vi "Main-RC.vi"() -> ()   [LabVIEW 2020]
uses:
  States.ctl
  <vilib>/measure/NI_MAPro.lvlib
  <vilib>/measure/matone.llb/Extract Single Tone Information 1 Chan.vi
  <vilib>/Analysis/NI_AALBase.lvlib
  <vilib>/Analysis/NI_AALPro.lvlib
  <vilib>/Analysis/6fits.llb/Confidence Interval (Exp).vi
  <vilib>/Analysis/baseanly.llb/Mean (DBL).vi
  <vilib>/DAQmx/read.llb/DAQmx Read (Analog 1D Wfm NChan NSamp).vi
  DAQmx_Parameters.ctl
  DAQmx_Channels.ctl
panel:
  in  "N_offset":i32 caption="last points"
  in  "Subtract":bool caption="Subtract mean of"
  out "DRC":dbl caption="us"
  out "RC=":dbl
  out "Fit XY Graph":cluster{dbl[], "Best Exponential Fit":dbl[]}[](graph) caption="Exponential Fit"
  in  "On/Off":bool
  in  "Fit Channel":u16(ring) caption="Analyse Channel" items=["Primo", "Secondo", "Terzo"]
  in  "ClearGraph":bool
  out "Freq Analisys":cluster{"X":dbl, "Y":dbl}[](graph) caption="Frequency Analysis"
  in  "Freq Chn":u16(ring) caption="Analyse Channel" items=["Primo", "Secondo", "Terzo"]
  out "data":waveform(dbl)[](graph) caption="DAQ Graphs"
  in  "DAQ Channels":T1=[{"DAQmx Physical"="", "Logic Name"="V_S", "Min Value"=-10.0, "Max Value"=10.0}, {"DAQmx Physical"="", "Logic Name"="V_C", "Min Value"=-10.0, "Max Value"=10.0}, {"DAQmx Physical"="", "Logic Name"="V_R", "Min Value"=-10.0, "Max Value"=10.0}]
  in  "DAQ Params":T2={"Trigger Level"=1.0, "Trigger Slope"=10280, "Sample Rate"=10000.0, "N Samples"=300} {"Trigger Slope" items=["Rising"=10280, "Falling"=10171]; "Trigger Level" scale=0.0..10.0}
  in  "FIT":bool caption="+ / -"
  in  "DAQ":bool
  in  "Stop":bool
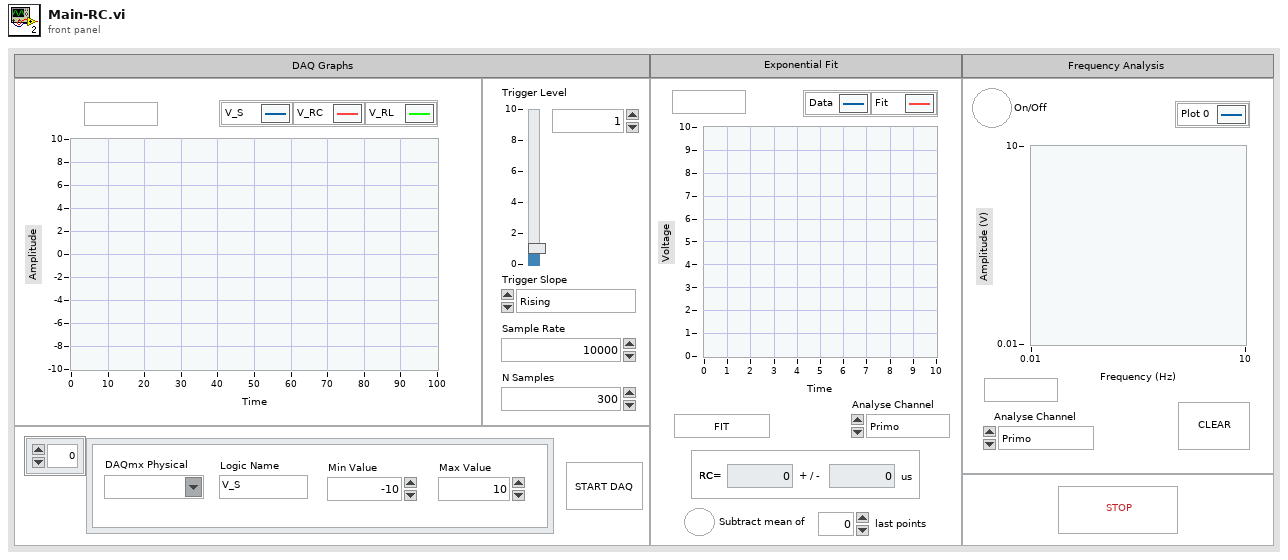
[diagram p1: front panel]
types:
  T1 = typedef "DAQmx_Channels.ctl" = cluster{"DAQmx Physical":tag, "Logic Name":string, "Min Value":dbl, "Max Value":dbl}[]
  T2 = typedef "DAQmx_Parameters.ctl" = cluster{"Trigger Level":dbl, "Trigger Slope":i32, "Sample Rate":dbl, "N Samples":i32}
  T3 = cluster{"detected frequency":dbl, "detected amplitude":dbl}[]
  T4 = typedef "States.ctl" = enum16{"Idle", "Acquire", "Fit", "Stop"}
  T5 = cluster{"detected frequency":dbl, "detected amplitude":dbl}
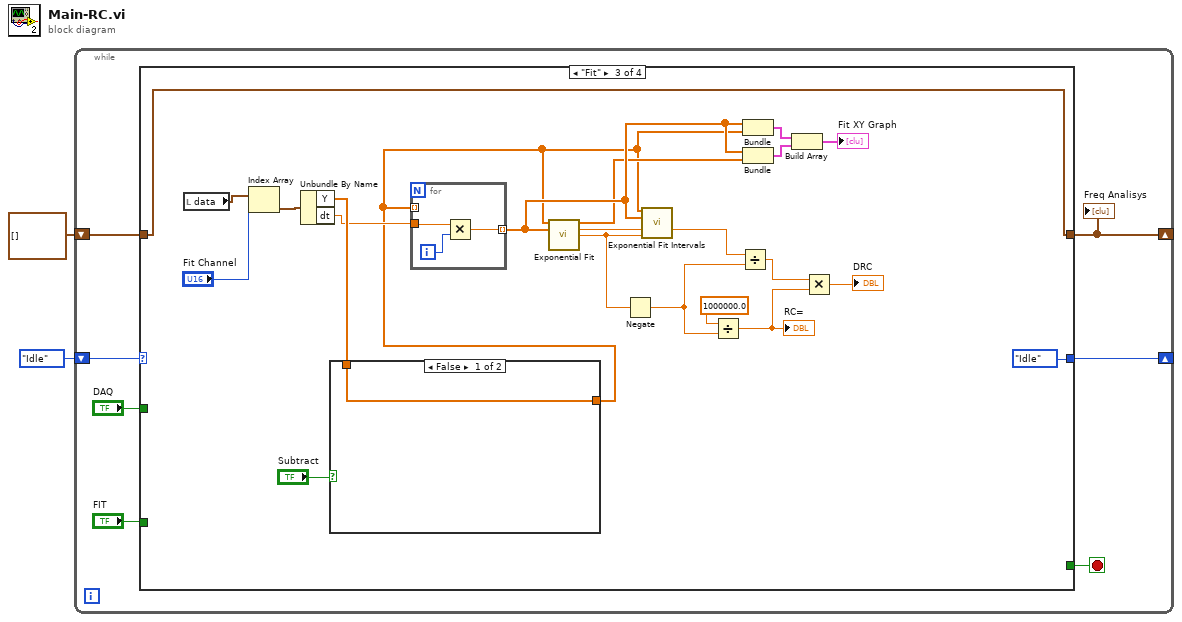
[diagram p0: block diagram]
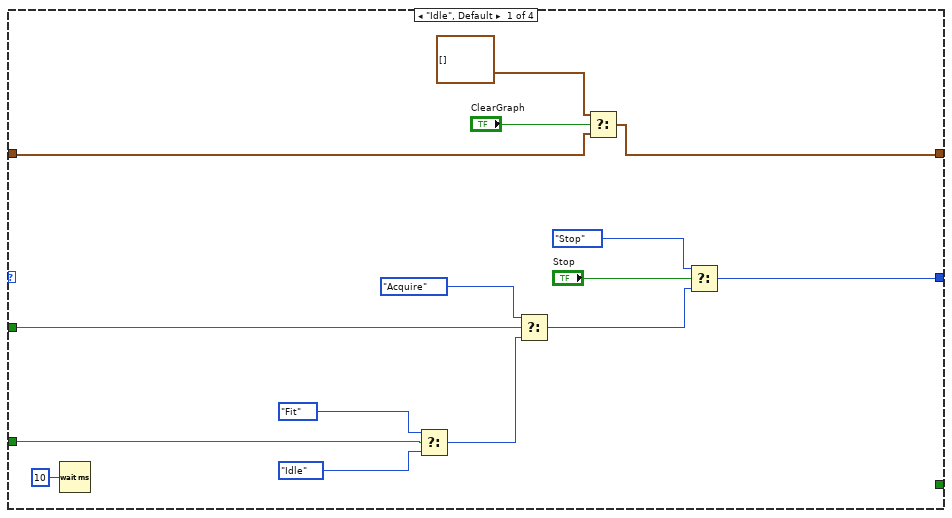
[diagram p2: hidden frame]
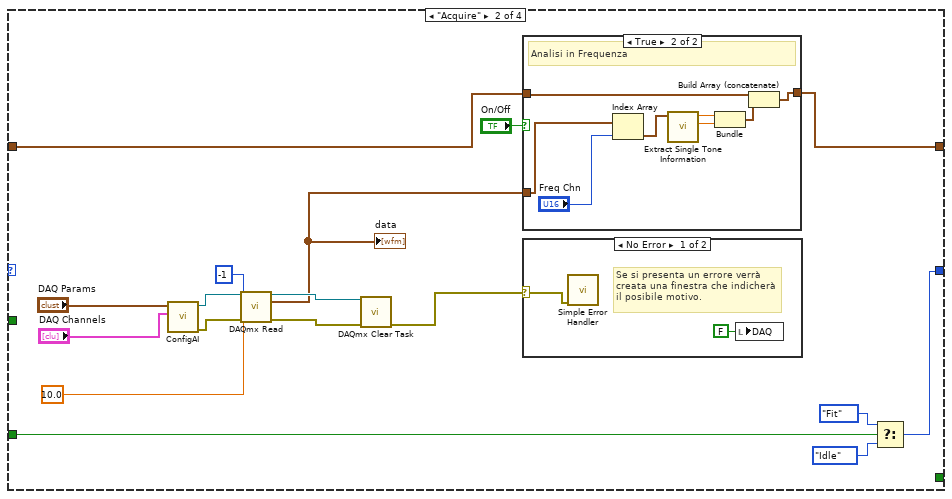
[diagram p3: hidden frame]
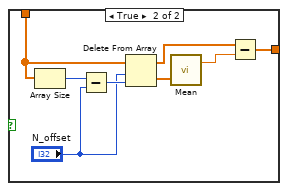
[diagram p6: hidden frame]
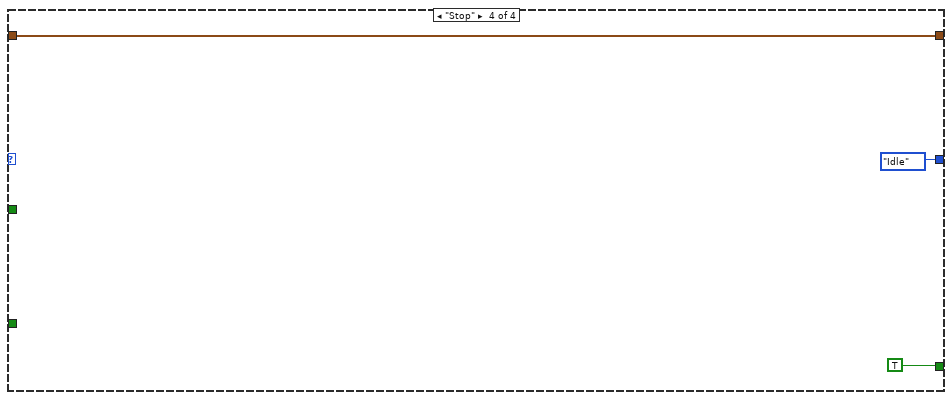
[diagram p7: hidden frame]
diagram:
  n1 = while {
    shift-right: [w7] -> _
    shift-left: States."Idle" ("Enum") -> [w9]
    shift-right: [w3] -> _
    shift-left: T3 [] -> [w4]
    stop <- w6 stop-if-true
    n2 = case shown="\"Fit\"" w9 {
      tunnel: "FIT" -> [w22 w34 _ _]
      tunnel: [w13 w40 States."Idle" ("Enum") States."Idle" ("Enum")] -> w7
      tunnel: [_ _ _ TRUE] -> w6
      tunnel: "DAQ" -> [w19 _ _ _]
      tunnel: w4 -> [w12 w37 w73 w88]
      tunnel: [w10 w36 w73 w88] -> w3
      frame "Idle", Default {
        n3 = Wait (ms)(milliseconds to wait=u32 10) -> ()  [unwired: 1 out]
        n4 = Select(t=States."Fit" ("Enum"), s=w22, f=States."Idle" ("Enum")) -> (s? t:f=w18:T4)
        n5 = Select(t=States."Acquire" ("Enum"), s=w19, f=w18) -> (s? t:f=w14:T4)
        n6 = Select(t=T3 [], s="ClearGraph", f=w12) -> (s? t:f=w10:T3)
        n7 = Select(t=States."Stop" ("Enum"), s="Stop", f=w14) -> (s? t:f=w13:T4)
      }
      frame "Acquire" {
        n8 = call "ConfigAI.vi"("DAQ Channels"="DAQ Channels", "DAQ Params"="DAQ Params") -> ("error out"=w32:errorcluster, "DAQmx Task Out"=w25:refnum<k21>)  [unwired: 8 in]
        n9 = call-poly <vilib>:"DAQmx Read.vi"("task/channels in"=w25, "number of samples per channel"=-1, "timeout"=10.0, "error in"=w32) -> ("task out"=w30:refnum<k21>, "data"=w27:waveform(dbl)[], "error out"=w29:errorcluster)  [unwired: 9 in]
        "data" <- w27
        n10 = call <vilib>:"DAQmx Clear Task.vi"("task in"=w30, "error in"=w29) -> ("error out"=w28:errorcluster)  [unwired: 13 in]
        n11 = case shown="True" "On/Off" {
          tunnel: w37 -> [w44 w49]
          tunnel: [w44 w48] -> w36
          tunnel: w27 -> [_ w45]
          frame False {
          }
          frame True {
            # "Analisi in Frequenza"
            n12 = Index Array(array=w45, index="Freq Chn") -> (element=w47:waveform(dbl))
            n13 = call-poly <vilib>:"Extract Single Tone Information.vi"("time signal in"=w47) -> ("detected amplitude"=w50:dbl, "detected frequency"=w51:dbl)  [unwired: 5 in, 4 out]
            n14 = Bundle("detected frequency"=w51, "detected amplitude"=w50) -> (w46:T5)  [unwired: 1 in]
            n15 = Build Array (concatenate)(w49, w46) -> (w48:T3)
          }
        }
        n16 = case shown="No Error" w28 {
          selector: w28 -> [w42 _]
          frame No Error {
            # "Se si presenta un errore verrà creata una finestra che indicherà il posibile motivo."
            n17 = call <vilib>:"Simple Error Handler.vi"("error in (no error)"=w42) -> ()  [unwired: 4 in, 5 out]
            n18 = local write "DAQ"(FALSE ("DAQ")) -> ()
          }
          frame Error {
          }
        }
        n19 = Select(t=States."Fit" ("Enum"), s=w34, f=States."Idle" ("Enum")) -> (s? t:f=w40:T4)
      }
      frame "Fit" {
        n20 = local read "data"() -> (w72:waveform(dbl)[])
        n21 = Index Array(array=w72, index="Fit Channel") -> (element=w53:waveform(dbl))
        n22 = Unbundle By Name(w53) -> ("Y"=w70:dbl[], "dt"=w68:dbl)
        n23 = case shown="False" "Subtract" {
          tunnel: w70 -> [w78 w85]
          tunnel: [w78 w79] -> w61
          frame False {
          }
          frame True {
            n24 = Array Size(array=w85) -> (size(s)=w86:i32)
            n25 = Subtract(x=w86, y="N_offset") -> (x-y=w84:i32)
            n26 = Delete From Array(array=w85, length="N_offset", index=w84) -> (deleted portion=w82:dbl[], array with subset deleted=w80:dbl[])
            n27 = call-poly <vilib>:"Mean.vi"("X"=w82) -> ("mean"=w81:dbl)  [unwired: 1 out]
            n28 = Subtract(x=w80, y=w81) -> (x-y=w79:dbl[])
          }
        }
        n29 = for {
          tunnel: w68 -> [w76]
          tunnel: [w75] -> w63 mode=indexing
          tunnel: w61 -> [_] mode=indexing
          i -> [w77]
          n30 = Multiply(x=w76, y=w77) -> (x*y=w75:dbl)
        }
        n31 = call <vilib>:"Exponential Fit.vi"("Y"=w61, "X"=w63) -> ("Best Exponential Fit"=w62:dbl[], "amplitude"=w65:dbl, "damping"=w59:dbl)  [unwired: 8 in, 3 out]
        n32 = Negate(x=w59) -> (-x=w57:dbl)
        n33 = call-poly <vilib>:"Exponential Fit Intervals.vi"("Y"=w61, "X"=w63, "amplitude"=w65, "damping"=w59) -> ("delta damping"=w60:dbl)  [unwired: 7 in, 4 out]
        n34 = Divide(x=1000000.0, y=w57) -> (x/y=w56:dbl)
        "RC=" <- w56
        n35 = Divide(x=w60, y=w57) -> (x/y=w55:dbl)
        n36 = Bundle(w63, "Y"=w61) -> (w67:cluster{dbl[], "Y":dbl[]})  [unwired: 1 in]
        n37 = Bundle(w63, "Best Exponential Fit"=w62) -> (w66:cluster{dbl[], "Best Exponential Fit":dbl[]})  [unwired: 1 in]
        n38 = Build Array(w67, w66) -> (→"Fit XY Graph":cluster{dbl[], "Best Exponential Fit":dbl[]}[])
        n39 = Multiply(x=w55, y=w56) -> (x*y=→"DRC":dbl)
      }
      frame "Stop" {
      }
    }
    "Freq Analisys" <- w3
  }
